vi "get_transformation_parameters.vi"(8 "error in (no error)":errorcluster, 11 "ScanHeadDL090202 in":refnum<class "ScanHeadDL090202.lvclass">) -> (0 "error out":errorcluster, 2 "transformation parameters":T1={"scale factor"=1.0, "rotation angle"=0.0, "tilting angle"=0.0, "offset"=refnum}, 3 "ScanHeadDL090202 out":refnum<class "ScanHeadDL090202.lvclass">)   [LabVIEW 2010, in "ScanHeadDL090202.lvclass"]
uses:
  ScanHeadDL090202.lvclass
  common/classes/SpaceVector/SpaceVector/SpaceVector.lvclass
  Trajectory/TrajectoryDL091126GenericVoxel/TrajectoryDL091126GenericVoxel/transformation_parameters.ctl
  Trajectory/TrajectoryDL091126GenericVoxel/TrajectoryDL091126GenericVoxel/TrajectoryDL091126GenericVoxel.lvclass
  common/classes/ErrorController/ErrorController/ErrorController.lvclass
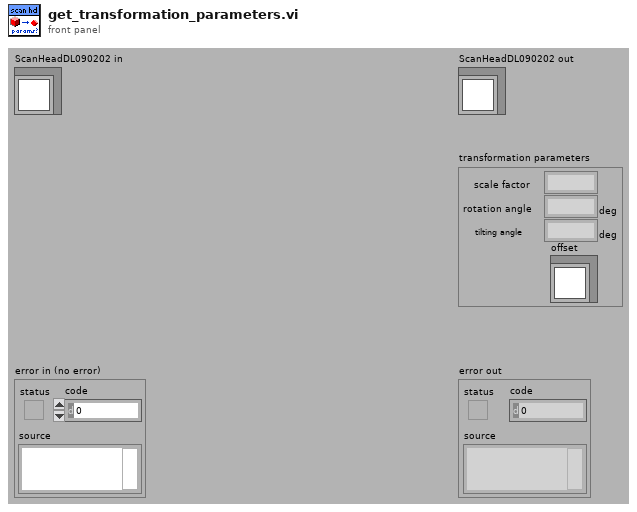
[diagram p1: front panel]
types:
  T1 = typedef "TrajectoryDL091126GenericVoxel.lvclass/transformation_parameters.ctl" = cluster{"scale factor":dbl, "rotation angle":dbl[unit], "tilting angle":dbl[unit], "offset":refnum<class "SpaceVector.lvclass">}
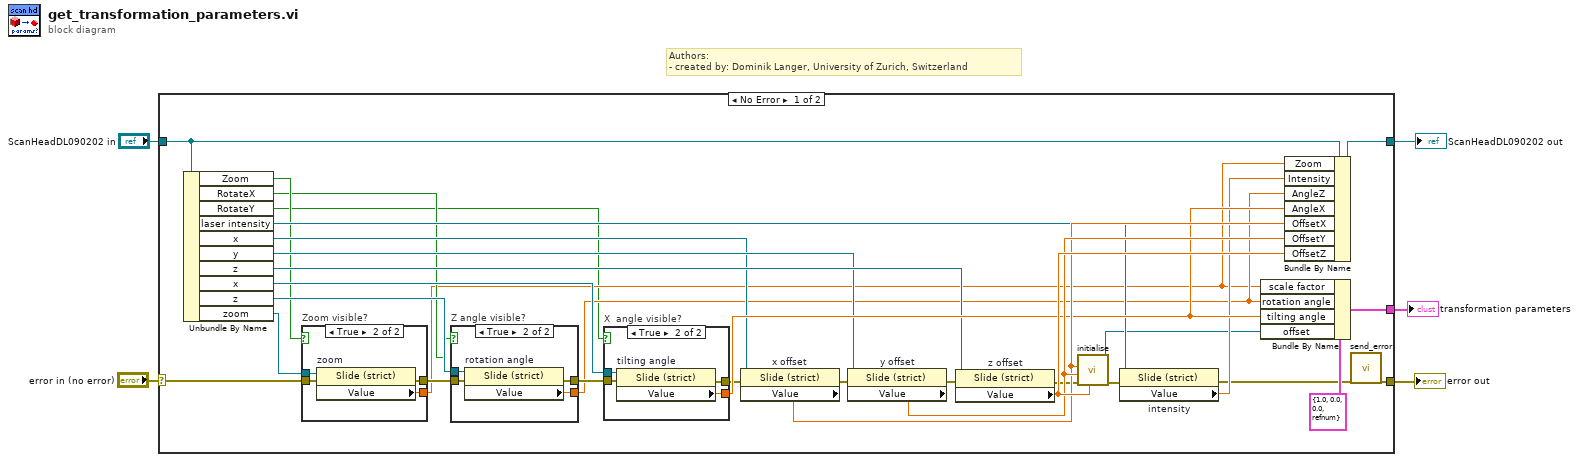
[diagram p0: block diagram]
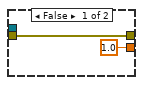
[diagram p4: hidden frame]
diagram:
  # "Authors: \n- created by: Dominik Langer, University of Zurich, Switzerland"
  n1 = case shown="No Error" "error in (no error)" {
    selector: "error in (no error)" -> [w18 w55]
    tunnel: [w10 w55] -> w4
    tunnel: [w12 w54] -> w2
    tunnel: "ScanHeadDL090202 in" -> [w13 w54]
    tunnel: [w16 _] -> w1
    frame No Error {
      n2 = Unbundle By Name(w13) -> ("Zoom"=w9:bool, "RotateX"=w8:bool, "RotateY"=w6:bool, "laser intensity"=w32:refnum<vi>, "x"=w27:refnum<vi>, "y"=w28:refnum<vi>, "z"=w29:refnum<vi>, "x"=w21:refnum<vi>, "z"=w20:refnum<vi>, "zoom"=w19:refnum<vi>)
      n3 = case "Zoom visible?" shown="True" w9 {
        tunnel: [1.0 ("Value") w53] -> w7
        tunnel: [w48 w52] -> w23
        tunnel: w19 -> [_ w51]
        tunnel: w18 -> [w48 w50]
        frame False {
        }
        frame True {
          n4 = property on="zoom" class="Slide (strict)"(reference=w51, error in=w50) -> (error out=w52:errorcluster, "Value"=w53:dbl)  [unwired: 1 out]
        }
      }
      n5 = case "Z angle visible?" shown="True" w8 {
        tunnel: w23 -> [w43 w47]
        tunnel: [w43 w46] -> w22
        tunnel: w20 -> [_ w45]
        tunnel: [_ w44] -> w14
        frame False {
        }
        frame True {
          n6 = property on="rotation angle" class="Slide (strict)"(reference=w45, error in=w47) -> (error out=w46:errorcluster, "Value"=w44:dbl[unit])  [unwired: 1 out]
        }
      }
      n7 = case "X  angle visible?" shown="True" w6 {
        tunnel: [_ w42] -> w34
        tunnel: [w38 w41] -> w24
        tunnel: w22 -> [w38 w40]
        tunnel: w21 -> [_ w39]
        frame False {
        }
        frame True {
          n8 = property on="tilting angle" class="Slide (strict)"(reference=w39, error in=w40) -> (error out=w41:errorcluster, "Value"=w42:dbl[unit])  [unwired: 1 out]
        }
      }
      n9 = property on="x offset" class="Slide (strict)"(reference=w27, error in=w24) -> (error out=w25:errorcluster, "Value"=w35:dbl[unit])  [unwired: 1 out]
      n10 = property on="y offset" class="Slide (strict)"(reference=w28, error in=w25) -> (error out=w26:errorcluster, "Value"=w36:dbl[unit])  [unwired: 1 out]
      n11 = property on="z offset" class="Slide (strict)"(reference=w29, error in=w26) -> (error out=w30:errorcluster, "Value"=w37:dbl[unit])  [unwired: 1 out]
      n12 = call "initialise.vi"("z"=w37, "error in (no error)"=w30, "y"=w36, "x"=w35) -> ("error out"=w17:errorcluster, "SpaceVector out"=w31:refnum<class "SpaceVector.lvclass">)  [unwired: 6 in]
      n13 = property on="intensity" class="Slide (strict)"(reference=w32, error in=w17) -> (error out=w11:errorcluster, "Value"=w33:dbl)  [unwired: 1 out]
      n14 = Bundle By Name(cluster=T1 {"scale factor"=1.0, "rotation angle"=0.0, "tilting angle"=0.0, "offset"=refnum} ("transformation parameters"), "scale factor"=w7, "rotation angle"=w14, "tilting angle"=w34, "offset"=w31) -> (w16:T1)
      n15 = Bundle By Name(cluster=w13, "Zoom"=w7, "Intensity"=w33, "AngleZ"=w14, "AngleX"=w34, "OffsetX"=w35, "OffsetY"=w36, "OffsetZ"=w37) -> (w12:refnum<class "ScanHeadDL090202.lvclass">)
      n16 = call "send_error.vi"("error in (no error)"=w11) -> ("error out"=w10:errorcluster)  [unwired: 10 in]
    }
    frame Error {
    }
  }
  "error out" <- w4
  "ScanHeadDL090202 out" <- w2
  "transformation parameters" <- w1
